vi "LaserControl.vi"() -> ()   [LabVIEW 2015]
doc: "An example of how you can get different types of images from the camera.\n\nNOTE: You must have ThermoVision installed to run this example."
uses:
  <userlib>/ThermoVision/ThermoVision Digital.llb/ThermoVision Digital ImageType.ctl
  <vilib>/Analysis/Matrix/NI_Matrix.lvlib
  <vilib>/Analysis/Matrix/Numeric/Conversions/Matrix To Array - RM.vi
  <userlib>/ThermoVision/ThermoVision.llb/Thermovision CameraTypes.ctl
  <userlib>/ThermoVision/ThermoVision.llb/ThermoVision DeviceTypes.ctl
  <userlib>/ThermoVision/ThermoVision.llb/ThermoVision CommunicationInterfaceType.ctl
  <userlib>/ThermoVision/ThermoVision Digital.llb/ThermoVision Digital ImageMode.ctl
panel:
  in  "Filter LBounds (C)":dbl
  in  "Filter UBounds (C)":dbl
  in  "HFV Driver COM (RS232)":refnum<visa-resource-name>
  in  "Flow Sensor COM (RS232)":refnum<visa-resource-name>
  in  "Duty Cycle":string
  out "Water Chiller Flow Sensor":bool
  out "COM Feed":string
  in  "Decrease Duty Cycle":bool
  in  "Increase Duty Cycle":bool
  in  "On":bool
  in  "HFV COM (RS232)":refnum<visa-resource-name>
  out "Probe4_Num":dbl
  out "Probe3_Num":dbl
  out "Probe2_Num":dbl
  out "Probe1_Num":dbl
  out "Probe 4":dbl(slide) scale=0.0..100.0
  out "Probe 3":dbl(slide) scale=0.0..100.0
  out "Probe 2":dbl(slide) scale=0.0..100.0
  out "Probe 1":dbl(slide) scale=0.0..100.0
  out "Thermometer":dbl(slide) scale=0.0..100.0
  in  "COM (RS232)":refnum<visa-resource-name>
  in  "Height Down":bool
  in  "Height Up":bool
  in  "Width Down":bool
  in  "Width Up":bool
  in  "Box Down":bool
  in  "Box Right":bool
  in  "Box Left":bool
  in  "Box Up":bool
  out "Camera":T1(plugin-control)
  out "Kelvin Multiplier":dbl=10.0
  out "Celsius":dbl
  out "Height":dbl=80.0
  out "Width":dbl=80.0
  out "Measure Box Y":dbl
  out "Measure Box X":dbl
  in  "Image Mode":T2=enum."Temperature (0.1K)"
  in  "Interface":T3=enum."UVC"
  in  "Device":T4=enum."USB video"
  in  "Camera Serial Number":string
  in  "CameraType":T5=enum."FLIR A615/A645/SC645/SC655"
  in  "error in (no error)":errorcluster
  in  "Stop":bool
  out "error out":errorcluster
  # "Selection Box Controls"
  # "Box Position"
  # "Box Width"
  # "Box Height"
  # "Measurement Filter"
  # "Fiber-Optic Probe Data"
  # "HFV-8000 Controls"
  # "Camera Interface"
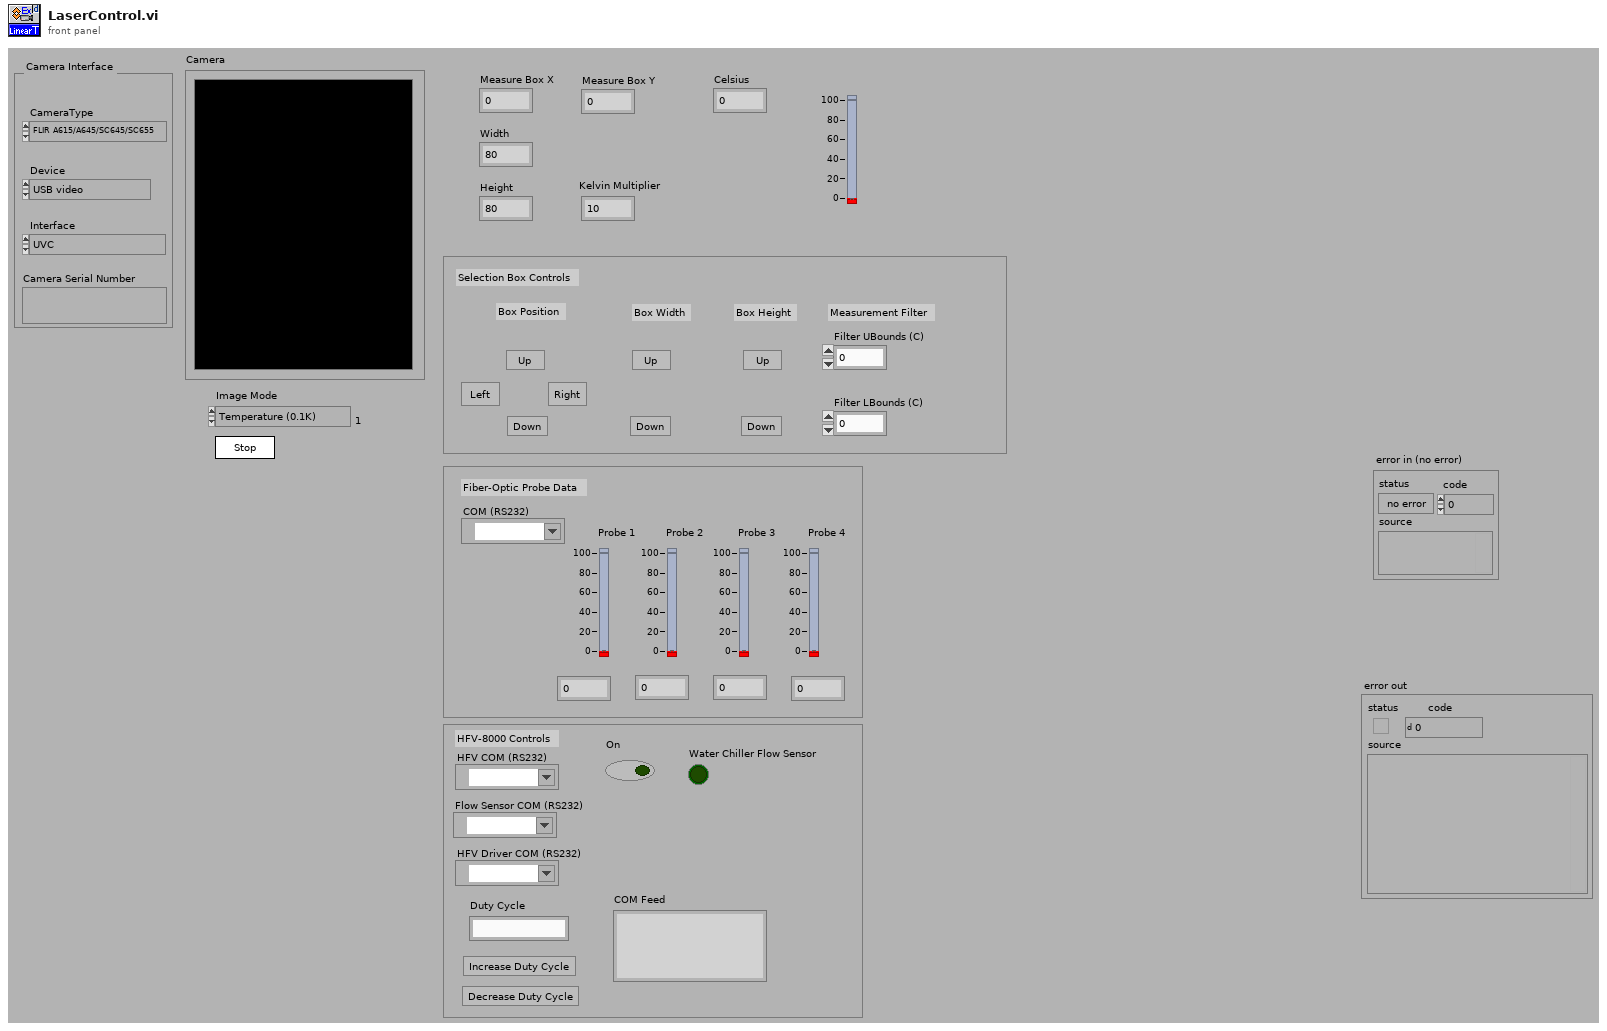
[diagram p1: front panel]
types:
  T1 = typedef "IMAQ Image.ctl" = refnum<image>
  T2 = typedef "ThermoVision Digital ImageMode.ctl" = enum16{"Signal", "Temperature (0.1K)", "Temperature (0.01K)"}
  T3 = typedef "ThermoVision CommunicationInterfaceType.ctl" = enum16{"File Only", "RS232", "TCP/IP(Ethernet)", "AV/C(FireWire)", "Gigabit Ethernet", "AXIS Video Server(Ethernet)", "UVC"}
  T4 = typedef "ThermoVision DeviceTypes.ctl" = enum16{"No Device", "FLIR PCCard", "ITEX IC-DIG 16", "Firewire 16-bit images", "Firewire 8-bit images", "Ethernet 16-bit images", "Ethernet 8-bit images", "IR-FlashLink", "iPort/GEV", "USB video"}
  T5 = typedef "Thermovision CameraTypes.ctl" = enum16{"ThermaCAM SC2000/SC3000", "THV 320/160", "ThermaCAM SC1000", "ThermaCAM S40/S45/S60/S65", "Thermovision A20/A40", "Cumulus SC4000/SC6000", "ThermaCAM SC640/SC660", "FLIR A320/A300/A310", "FLIR A325(A320G)/A315/SC305/SC325", "Indigo Merlin", "Indigo Phoenix", "Indigo Omega", "THV 1000", "THV 900", "FLIR GF320/GF309", "FLIR T-series", "FLIR A615/A645/SC645/SC655", "FLIR Exx series", "FLIR T620/T640/T420/T440"}
  T6 = enum16{"Internal Image Correction", "External Image Correction", "Auto Adjust", "Show Camera Info Dialog", "Show Device Status Dialog", "Reload Calibration(SC1000 only)"}
  T7 = enum16{"Unused0", "Unused1", "Unused2", "Unused3", "Unused4", "Unused5", "Unused6", "U16 Grayscale"}
  T8 = typedef "ThermoVision Digital ImageType.ctl" = enum16{"Raw", "Absolute", "Object", "Temperature", "Raw 8 bits"}
  T9 = typedef "Thermovision Object Reference.ctl" = refnum<k1>
  T10 = cluster{"Measure Box X":dbl, "Measure Box Y":dbl, dbl, dbl}
  T11 = typedef "LVPoint32TypeDef.ctl" = cluster{"Horizontal":i32, "Vertical":i32}
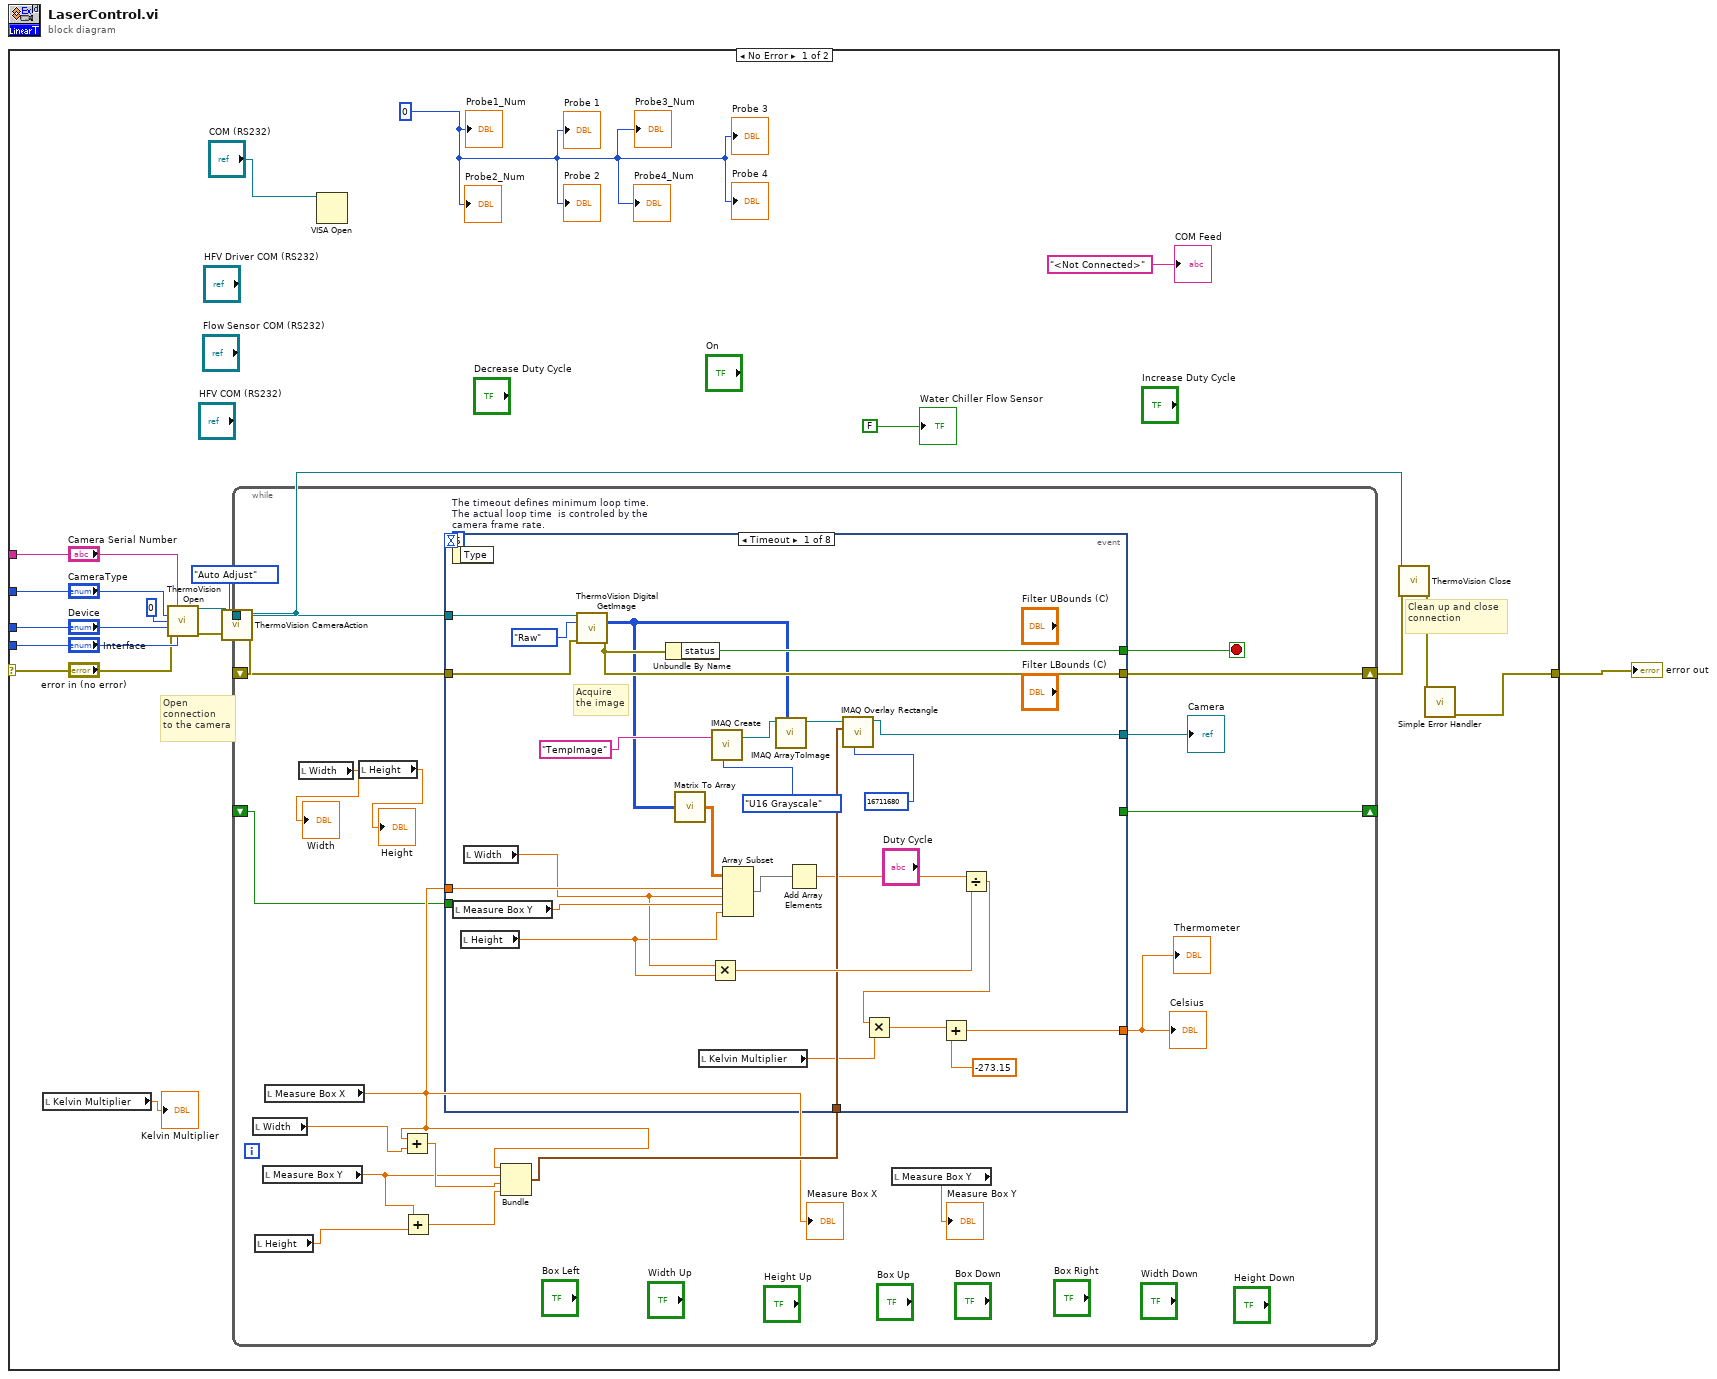
[diagram p0: block diagram]
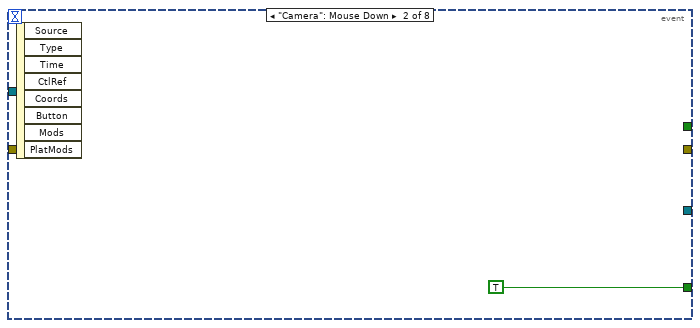
[diagram p2: hidden frame]
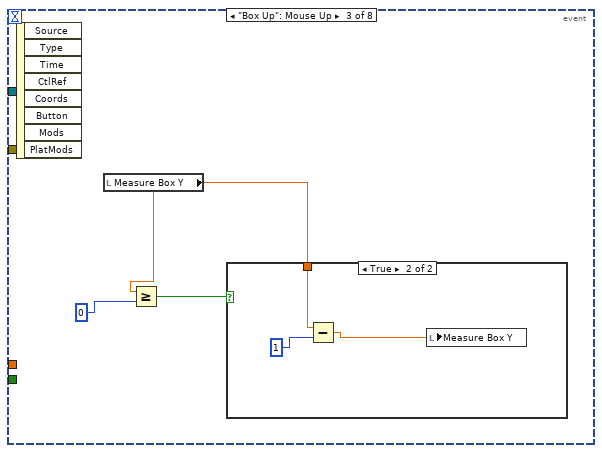
[diagram p3: hidden frame]
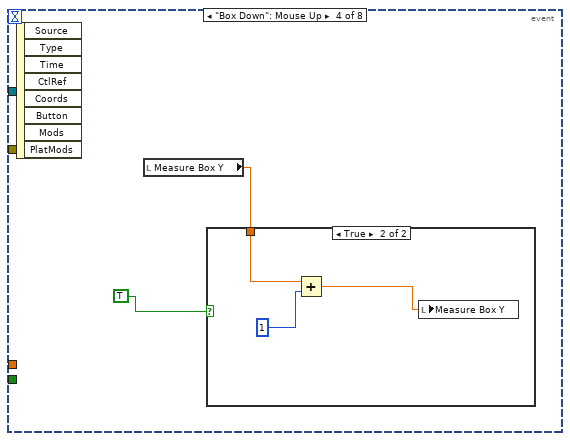
[diagram p5: hidden frame]
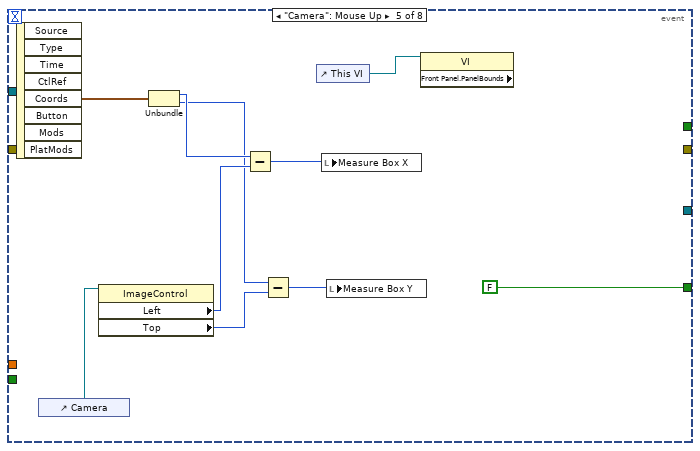
[diagram p7: hidden frame]
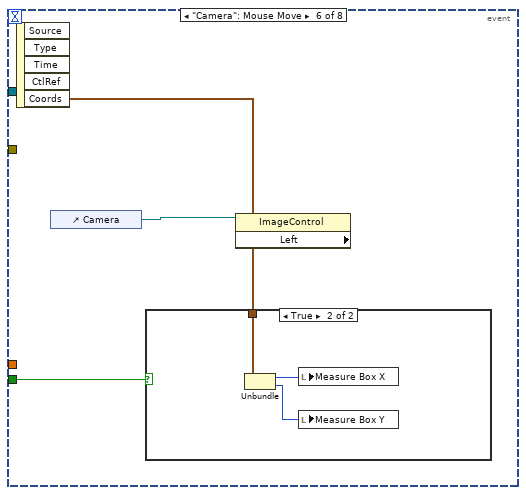
[diagram p8: hidden frame]
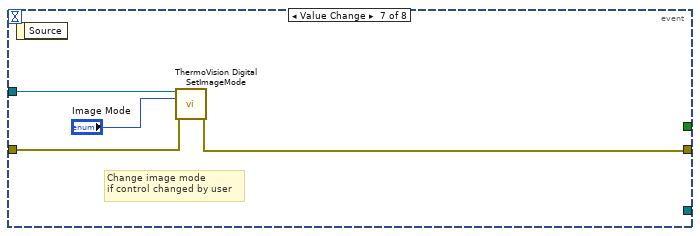
[diagram p10: hidden frame]
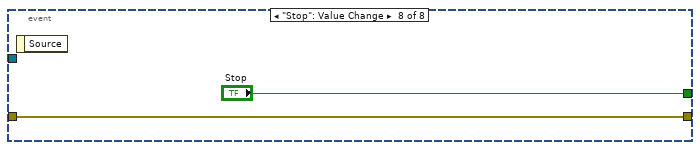
[diagram p11: hidden frame]
diagram:
  n1 = case shown="No Error" "error in (no error)" {
    selector: "error in (no error)" -> [w12 w105]
    tunnel: "CameraType" -> [w25 _]
    tunnel: [w23 w105] -> w5
    tunnel: "Camera Serial Number" -> [w21 _]
    tunnel: "Device" -> [w20 _]
    tunnel: "Interface" -> [w19 _]
    frame No Error {
      w9 = 0
      # "Open \nconnection\nto the camera"
      # "Clean up and close\nconnection"
      n2 = local read "Kelvin Multiplier"() -> (→"Kelvin Multiplier":dbl)
      n3 = call <userlib>:"ThermoVision Open.vi"("Server/SN"=w21, "CameraType"=w25, "Port"=i16 0, "Device"=w20, "error in (no error)"=w12, "Interface"=w19) -> ("reference"=w18:T9, "error out"=w16:errorcluster)  [unwired: 8 in]
      n4 = call <userlib>:"ThermoVision CameraAction.vi"("error in (no error)"=w16, "Action"=T6."Auto Adjust", "reference"=w18) -> ("error out"=w14:errorcluster, "duplicate reference"=w17:T9)  [unwired: 7 in]
      n5 = while {
        shift-right: [w43] -> w13
        shift-left: w14 -> [w42]
        tunnel: w17 -> [w44]
        shift-right: [w36] -> _
        shift-left: _ -> [w28]
        stop <- w40 stop-if-true
        w41 = 5  # The timeout defines minimum loop time.  The actual loop time  is controled by the camera frame rate.
        n6 = local read "Width"() -> (w30:dbl)
        n7 = local read "Height"() -> (w29:dbl)
        n8 = local read "Measure Box Y"() -> (w31:dbl)
        n9 = local read "Measure Box X"() -> (w35:dbl)
        "Measure Box X" <- w35
        n10 = local read "Width"() -> (→"Width":dbl)
        n11 = local read "Height"() -> (→"Height":dbl)
        n12 = Add(x=w35, y=w30) -> (x+y=w37:dbl)
        n13 = Add(x=w31, y=w29) -> (x+y=w39:dbl)
        n14 = Bundle("Measure Box X"=w35, "Measure Box Y"=w31, w37, w39) -> (w38:T10)  [unwired: 1 in]
        n15 = event shown="[0] Timeout" {
          selector: _ -> [_ _ _ _ _ _ _ _]
          dyn-events: _ -> [_ _ _ _ _ _ _ _]
          timeout: w41 -> [_ _ _ _ _ _ _ _]
          tunnel: w42 -> [w66 _ _ _ _ _ w102 w103]
          tunnel: w44 -> [w69 _ _ _ _ _ w101 _]
          tunnel: [w68 _ _ _ _ _ w100 w103] -> w43
          tunnel: [w67 _ _ _ _ _ _ "Stop"] -> w40
          tunnel: w35 -> [w61 _ _ _ _ _ _ _]
          tunnel: w38 -> [w59 _ _ _ _ _ _ _]
          tunnel: [w52 _ _ _ _ _ _ _] -> w27
          tunnel: [_ TRUE _ _ FALSE _ _ _] -> w36
          tunnel: w28 -> [_ _ _ _ _ w95 _ _]
          tunnel: [w45 _ _ _ _ _ _ _] -> w26
          event Timeout {
            # "Acquire\nthe image"
            n16 = event-data() -> ()  [unwired: 1 in, 1 out]
            n17 = local read "Measure Box Y"() -> (w50:dbl)
            n18 = local read "Height"() -> (w47:dbl)
            n19 = local read "Width"() -> (w48:dbl)
            n20 = call <userlib>:"ThermoVision Digital GetImage.vi"("reference"=w69, "ImageType"=ThermoVision_Digital_ImageType."Raw", "error in (no error)"=w66) -> ("Image(U16)"=w54:u16[][], "error out"=w68:errorcluster)  [unwired: 7 in, 4 out]
            n21 = Unbundle By Name(w68) -> ("status"=w67:bool)
            n22 = call-poly <vilib>:"Matrix To Array.vi"("Real Matrix"=w54) -> ("Real 2D Array"=w60:dbl[][])
            n23 = local read "Kelvin Multiplier"() -> (w49:dbl)
            n24 = Multiply(x=w48, y=w47) -> (x*y=w64:dbl)
            n25 = call "IMAQ Create"("Image Name"="TempImage", "Image Type"=T7."U16 Grayscale") -> ("New Image"=w57:T1)  [unwired: 3 in, 1 out]
            n26 = Array Subset(array=w60, index (row)=w61, length (row)=w48, index (col)=w50, length (col)=w47) -> (w65:dbl[][])
            n27 = call "IMAQ ArrayToImage"("Image Pixels (U16)"=w54, "Image"=w57) -> ("Image Out"=w58:T1)  [unwired: 8 in, 1 out]
            n28 = Add Array Elements(numeric array=w65) -> (sum=w46:dbl)
            n29 = call "IMAQ Overlay Rectangle"("Color"=16711680, "Rectangle"=w59, "Image"=w58) -> ("Image Out"=w45:T1)  [unwired: 7 in, 1 out]
            n30 = Divide(x=w46, y=w64) -> (x/y=w51:dbl)
            n31 = Multiply(x=w51, y=w49) -> (x*y=w63:dbl)
            n32 = Add(x=w63, y=-273.15) -> (x+y=w52:dbl)
          }
          event "Camera": Mouse Down {
            n33 = event-data() -> ()  [unwired: 1 in, 8 out]
          }
          event "Box Up": Mouse Up {
            n34 = event-data() -> ()  [unwired: 1 in, 8 out]
            n35 = local read "Measure Box Y"() -> (w72:dbl)
            n36 = Greater Or Equal?(x=w72, y=0) -> (x >= y?=w73:bool)
            n37 = case shown="True" w73 {
              tunnel: w72 -> [_ w76]
              frame False {
              }
              frame True {
                n38 = Subtract(x=w76, y=1) -> (x-y=w77:dbl)
                n39 = local write "Measure Box Y"(w77) -> ()
              }
            }
          }
          event "Box Down": Mouse Up {
            n40 = event-data() -> ()  [unwired: 1 in, 8 out]
            n41 = local read "Measure Box Y"() -> (w78:dbl)
            n42 = case shown="True" TRUE {
              tunnel: w78 -> [_ w81]
              frame False {
              }
              frame True {
                n43 = Add(x=w81, y=1) -> (x+y=w80:dbl)
                n44 = local write "Measure Box Y"(w80) -> ()
              }
            }
          }
          event "Camera": Mouse Up {
            n45 = event-data() -> ("Coords"=w83:T11)  [unwired: 1 in, 7 out]
            n46 = control-ref of="Camera"() -> (w85:refnum<vi>)
            n47 = property class="ImageControl"(reference=w85) -> ("Left"=w91:i32, "Top"=w87:i32)  [unwired: 1 in, 2 out]
            n48 = Unbundle(w83) -> ("Horizontal"=w90:i32, "Vertical"=w88:i32)
            n49 = Subtract(x=w90, y=w91) -> (x-y=w89:i32)
            n50 = Subtract(x=w88, y=w87) -> (x-y=w86:i32)
            n51 = control-ref of="This VI"() -> (w84:refnum<vi>)
            n52 = local write "Measure Box X"(w89) -> ()
            n53 = local write "Measure Box Y"(w86) -> ()
            n54 = property class="VI" props=["Front Panel.PanelBounds"](reference=w84) -> ()  [unwired: 1 in, 3 out]
          }
          event "Camera": Mouse Move {
            n55 = event-data() -> ("Coords"=w94:T11)  [unwired: 1 in, 4 out]
            n56 = control-ref of="Camera"() -> (w93:refnum<vi>)
            n57 = case shown="True" w95 {
              tunnel: w94 -> [_ w96]
              frame False {
              }
              frame True {
                n58 = Unbundle(w96) -> ("Horizontal"=w97:i32, "Vertical"=w98:i32)
                n59 = local write "Measure Box X"(w97) -> ()
                n60 = local write "Measure Box Y"(w98) -> ()
              }
            }
            n61 = property class="ImageControl" props=["Left"](reference=w93) -> ()  [unwired: 1 in, 3 out]
          }
          event Value Change {
            # "Change image mode\nif control changed by user"
            n62 = event-data() -> ()  [unwired: 1 in, 1 out]
            n63 = call <userlib>:"ThermoVision Digital SetImageMode.vi"("reference"=w101, "Image Mode"="Image Mode", "error in (no error)"=w102) -> ("error out"=w100:errorcluster)  [unwired: 11 in, 1 out]
          }
          event "Stop": Value Change {
            n64 = event-data() -> ()  [unwired: 1 in, 1 out]
          }
        }
        "Celsius" <- w27
        "Thermometer" <- w27
        "Camera" <- w26
        n65 = local read "Measure Box Y"() -> (→"Measure Box Y":dbl)
      }
      n66 = VISA Open(VISA resource name="COM (RS232)") -> ()  [unwired: 4 in, 2 out]
      n67 = call <userlib>:"ThermoVision Close.vi"("reference"=w17, "error in (no error)"=w13) -> ("error out"=w24:errorcluster)  [unwired: 13 in]
      n68 = call <vilib>:"Simple Error Handler.vi"("error in (no error)"=w24) -> ("error out"=w23:errorcluster)  [unwired: 4 in, 4 out]
      "Probe1_Num" <- w9
      "Probe2_Num" <- w9
      "Probe3_Num" <- w9
      "Water Chiller Flow Sensor" <- FALSE
      "Probe 1" <- w9
      "Probe 2" <- w9
      "Probe 3" <- w9
      "Probe 4" <- w9
      "Probe4_Num" <- w9
      "COM Feed" <- "<Not Connected>"
    }
    frame Error {
    }
  }
  "error out" <- w5
